vi "Receive Message.vi"(6 "priority":i32, 10 "Instrument Owner in":refnum<class "Instrument Owner.lvclass">, 11 "Message in":refnum<class "Message.lvclass">) -> (0 "error out":errorcluster, 2 "Actor out":refnum<class "Actor.lvclass">)   [LabVIEW 2020, in "Instrument Handler.lvlib" / "Instrument Owner.lvclass"]
doc: "Forward Instrument Msg classes to the Instrument sequencer after Sync Locking."
uses:
  Instrument Owner.lvclass
  PPL/HDH.Actor Framework.Core.Actor.lvlibp/1abvi3w/vi.lib/ActorFramework/Message/Message.lvclass
  PPL/HDH.Actor Framework.Core.Actor.lvlibp/1abvi3w/vi.lib/ActorFramework/Actor/Actor.lvclass
  C:/Current projects/WS/PPL/HDH.Actor Framework.Core.Actor.lvlibp/1abvi3w/vi.lib/ActorFramework/Actor/Actor.lvclass
  Messages/Instrument Msg/Instrument Msg.lvclass
  C:/Current projects/WS/PPL/HDH.Actor Framework.Core.Actor.lvlibp/1abvi3w/vi.lib/ActorFramework/Message/Message.lvclass
  PPL/HDH.Actor Framework.Core.Sequencer.lvlibp/Sequencer/Sequencer.lvclass
  PPL/HDH.Actor Framework.Core.Publisher.lvlibp/Messages/Response Msg/Response Msg.lvclass
  C:/Current projects/WS/PPL/HDH.Actor Framework.Core.Publisher.lvlibp/Messages/Response Msg/Response Msg.lvclass
  C:/Current projects/WS/PPL/HDH.Actor Framework.Core.Sequencer.lvlibp/Sequencer/Sequencer.lvclass
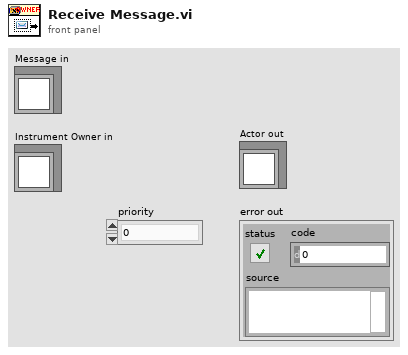
[diagram p1: front panel]
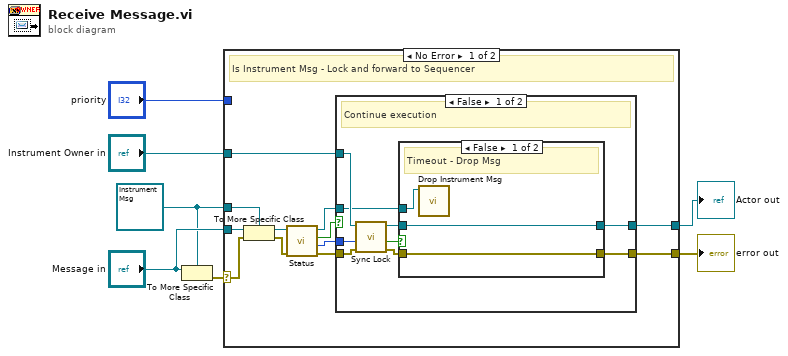
[diagram p0: block diagram]
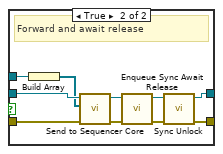
[diagram p2: hidden frame]
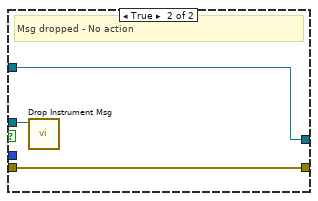
[diagram p3: hidden frame]
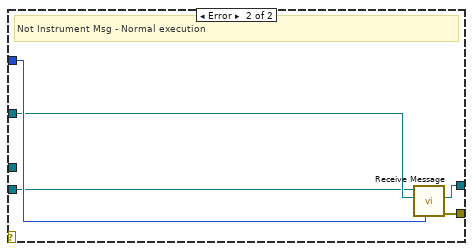
[diagram p4: hidden frame]
diagram:
  w1 = refnum<class "Instrument Msg.lvclass"> refnum ("Instrument Handler.lvlib:Instrument Msg.lvclass")
  n1 = To More Specific Class(target class=w1, reference="Message in") -> (error out=w3:errorcluster)  [unwired: 1 in, 1 out]
  n2 = case shown="No Error" w3 {
    selector: w3 -> [w19 _]
    tunnel: [w14 w49] -> w7
    tunnel: [w15 w48] -> w6
    tunnel: "priority" -> [_ w47]
    tunnel: "Instrument Owner in" -> [w16 w46]
    tunnel: "Message in" -> [w18 w45]
    tunnel: w1 -> [w17 _]
    frame No Error {
      # "Is Instrument Msg - Lock and forward to Sequencer"
      n3 = To More Specific Class(target class=w17, reference=w18, error in=w19) -> (specific class reference=w13:refnum<class "Instrument Msg.lvclass">, error out=w11:errorcluster)
      n4 = call "Status.vi"("error in (no error)"=w11, "Response Msg in"=w13) -> ("error out"=w10:errorcluster, "Time to Timeout (ms)"=w8:i32, "Dropped?"=w9:bool, "Response Msg out"=w12:refnum<class "Instrument Msg.lvclass">)  [unwired: 6 in]
      n5 = case shown="False" w9 {
        tunnel: w16 -> [w28 w44]
        tunnel: [w24 w44] -> w15
        tunnel: [w23 w42] -> w14
        tunnel: w12 -> [w22 w43]
        tunnel: w10 -> [w21 w42]
        tunnel: w8 -> [w20 _]
        frame False {
          # "Continue execution"
          n6 = call "Sync Lock.vi"("error in (no error)"=w21, "Timeout (-1ms)"=w20, "Instrument Owner in"=w28) -> ("error out"=w26:errorcluster, "Success?"=w25:bool, "Instrument Owner out"=w27:refnum<class "Instrument Owner.lvclass">)  [unwired: 6 in]
          n7 = case shown="False" w25 {
            tunnel: w27 -> [w31 w41]
            tunnel: w26 -> [w29 w40]
            tunnel: w22 -> [w30 w39]
            tunnel: [w31 w33] -> w24
            tunnel: [w29 w32] -> w23
            frame False {
              # "Timeout - Drop Msg"
              n8 = call "Drop Instrument Msg.vi"("Instrument Msg in"=w30) -> ()  [unwired: 11 in]
            }
            frame True {
              # "Forward and await release"
              n9 = Build Array(w39) -> (w38:refnum<class "Instrument Msg.lvclass">[])
              n10 = call "Send to Sequencer Core.vi"("error in (no error)"=w40, "Message Array"=w38, "Sequencer in"=w41) -> ("error out"=w36:errorcluster, "Sequencer out"=w37:refnum<class "Instrument Owner.lvclass">)  [unwired: 7 in]
              n11 = call "Enqueue Sync Await Release.vi"("error in (no error)"=w36, "Instrument Owner in"=w37) -> ("error out"=w34:errorcluster, "Instrument Owner out"=w35:refnum<class "Instrument Owner.lvclass">)  [unwired: 8 in]
              n12 = call "Sync Unlock.vi"("error in (no error)"=w34, "Instrument Owner in"=w35) -> ("error out"=w32:errorcluster, "Instrument Owner out"=w33:refnum<class "Instrument Owner.lvclass">)  [unwired: 8 in]
            }
          }
        }
        frame True {
          # "Msg dropped - No action"
          n13 = call "Drop Instrument Msg.vi"("Instrument Msg in"=w43) -> ()  [unwired: 11 in]
        }
      }
    }
    frame Error {
      # "Not Instrument Msg - Normal execution"
      n14 = call-parent "Receive Message.vi"("priority"=w47, "Sequencer in"=w46, "Message in"=w45) -> ("error out"=w49:errorcluster, "Actor out"=w48:refnum<class "Actor.lvclass">)  [unwired: 7 in]
    }
  }
  "error out" <- w7
  "Actor out" <- w6
